vi "Create.vi"(8 "Error In":errorcluster, 10 "Tag":string, 11 "Display Element In":refnum<class "Display Element.lvclass">) -> (0 "Error Out":errorcluster, 3 "Display Element":refnum<class "Display Element.lvclass">)   [LabVIEW 2019, in "Display Element.lvclass"]
uses:
  Display Element.lvclass
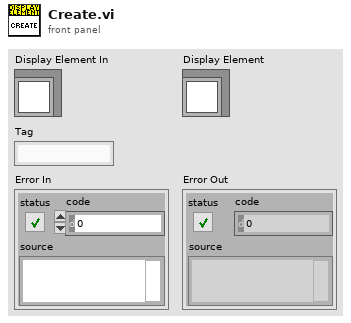
[diagram p1: front panel]
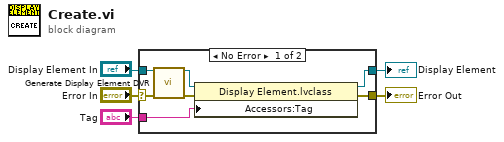
[diagram p0: block diagram]
diagram:
  n1 = case shown="No Error" "Error In" {
    selector: "Error In" -> [w12 w14]
    tunnel: [w7 w14] -> w4
    tunnel: [w8 w13] -> w3
    tunnel: "Display Element In" -> [w11 w13]
    tunnel: "Tag" -> [w6 _]
    frame No Error {
      n2 = call "Generate Display Element DVR.vi"("Error In"=w12, "Display Element In"=w11) -> ("Error Out"=w9:errorcluster, "Display Element Out"=w10:refnum<class "Display Element.lvclass">)  [unwired: 8 in]
      n3 = property class="Display Element.lvclass"(reference=w10, error in=w9, "Accessors:Tag"=w6) -> (reference out=w8:refnum<class "Display Element.lvclass">, error out=w7:errorcluster)
    }
    frame Error {
    }
  }
  "Display Element" <- w3
  "Error Out" <- w4
